vi "process_shutter.vi"(6 "error in (no error)":errorcluster) -> (0 "error out":errorcluster)   [LabVIEW 2010]
uses:
  typedefs/control_shutter_enum.ctl
  <vilib>/DAQmx/write.llb/DAQmx Write (Digital Bool 1Line 1Point).vi
  <vilib>/DAQmx/create/channels.llb/DAQmx Create Channel (DO-Digital Output).vi
  <vilib>/daqmx/miscellaneous.llb/DAQmx Fill In Error Info.vi
panel:
  out "Shutter":bool
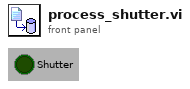
[diagram p1: front panel]
types:
  T1 = typedef "control_shutter_enum.ctl" = enum16{"Init", "Open", "Close", "Quit"}
  T2 = cluster{"Control shutter enum":T1, "variant":variant}
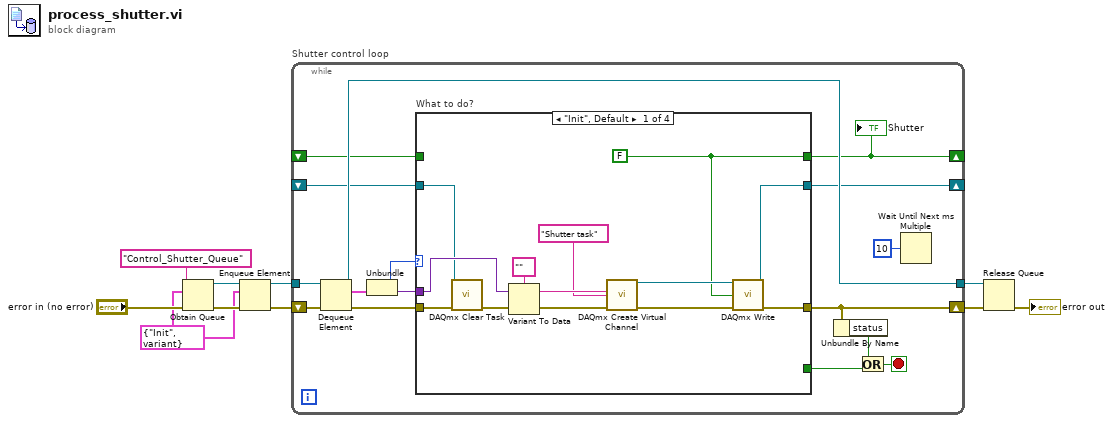
[diagram p0: block diagram]
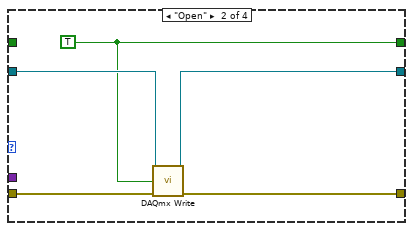
[diagram p2: hidden frame]
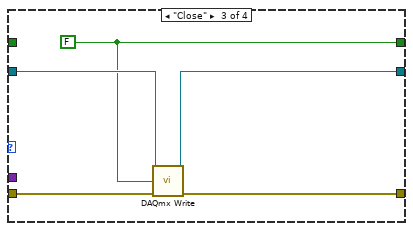
[diagram p3: hidden frame]
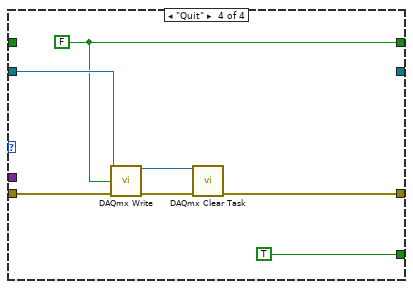
[diagram p4: hidden frame]
diagram:
  w3 = T2 {"Control shutter enum"=enum."Init", "variant"=variant}
  n1 = Obtain Queue(name (unnamed)="Control_Shutter_Queue", element data type=w3, error in (no error)="error in (no error)") -> (queue out=w6:refnum<queue>, error out=w4:errorcluster)  [unwired: 2 in, 1 out]
  n2 = Enqueue Element(queue=w6, element=w3, error in (no error)=w4) -> (queue out=w5:refnum<queue>, error out=w2:errorcluster)  [unwired: 1 in, 1 out]
  n3 = while "Shutter control loop" {
    shift-right: [w20] -> w1
    shift-left: w2 -> [w25]
    tunnel: w5 -> [w26]
    tunnel: [w16] -> w7
    shift-right: [w14] -> _
    shift-left: _ -> [w13]
    shift-right: [w12] -> _
    shift-left: _ -> [w11]
    stop <- w18 stop-if-true
    n4 = Dequeue Element(queue=w26, error in (no error)=w25) -> (queue out=w16:refnum<queue>, element=w24:T2, error out=w21:errorcluster)  [unwired: 1 in, 1 out]
    n5 = Unbundle(w24) -> ("Control shutter enum"=w23:T1, "variant"=w22:variant)
    n6 = case "What to do?" shown="\"Init\", Default" w23 {
      tunnel: w22 -> [w39 _ _ _]
      tunnel: w21 -> [w29 w41 w46 w54]
      tunnel: [w33 w44 w49 w55] -> w20
      tunnel: [_ _ _ TRUE] -> w17
      tunnel: [w31 w40 w45 _] -> w14
      tunnel: w13 -> [w27 w43 w48 w52]
      tunnel: [w30 w42 w47 w50] -> w12
      tunnel: w11 -> [_ _ _ _]
      frame "Init", Default {
        w30 = FALSE ("data")
        n7 = call <vilib>:"DAQmx Clear Task.vi"("task in"=w27, "error in"=w29) -> ("error out"=w28:errorcluster)  [unwired: 13 in]
        n8 = Variant To Data(error in=w28, Variant=w39, type=tag "" ("lines")) -> (error out=w38:errorcluster, data=w36:tag)
        n9 = call-poly <vilib>:"DAQmx Create Virtual Channel.vi"("lines"=w36, "name to assign"="Shutter task", "error in"=w38) -> ("task out"=w32:refnum<k21>, "error out"=w34:errorcluster)  [unwired: 11 in]
        n10 = call-poly <vilib>:"DAQmx Write.vi"("task/channels in"=w32, "data"=w30, "error in"=w34) -> ("task out"=w31:refnum<k21>, "error out"=w33:errorcluster)  [unwired: 10 in, 1 out]
      }
      frame "Open" {
        w42 = TRUE
        n11 = call-poly <vilib>:"DAQmx Write.vi"("task/channels in"=w43, "data"=w42, "error in"=w41) -> ("task out"=w40:refnum<k21>, "error out"=w44:errorcluster)  [unwired: 10 in, 1 out]
      }
      frame "Close" {
        w47 = FALSE
        n12 = call-poly <vilib>:"DAQmx Write.vi"("task/channels in"=w48, "data"=w47, "error in"=w46) -> ("task out"=w45:refnum<k21>, "error out"=w49:errorcluster)  [unwired: 10 in, 1 out]
      }
      frame "Quit" {
        w50 = FALSE ("data")
        n13 = call-poly <vilib>:"DAQmx Write.vi"("task/channels in"=w52, "data"=w50, "error in"=w54) -> ("task out"=w51:refnum<k21>, "error out"=w53:errorcluster)  [unwired: 10 in, 1 out]
        n14 = call <vilib>:"DAQmx Clear Task.vi"("task in"=w51, "error in"=w53) -> ("error out"=w55:errorcluster)  [unwired: 13 in]
      }
    }
    "Shutter" <- w12
    n15 = Unbundle By Name(w20) -> ("status"=w19:bool)
    n16 = Or(x=w19, y=w17) -> (x .or. y?=w18:bool)
    n17 = Wait Until Next ms Multiple(millisecond multiple=u32 10) -> ()  [unwired: 1 out]
  }
  n18 = Release Queue(queue=w7, error in (no error)=w1) -> (error out=→"error out":errorcluster)  [unwired: 1 in, 2 out]
